vi "Model--Set Value.vi"(8 "error in":errorcluster, 10 "Value":i32, 11 "Selector in":refnum<class "Selector.lvclass">) -> (0 "error out":errorcluster, 3 "Selector out":refnum<class "Selector.lvclass">)   [LabVIEW 2019, in "Selector.lvclass"]
uses:
  Selector.lvclass
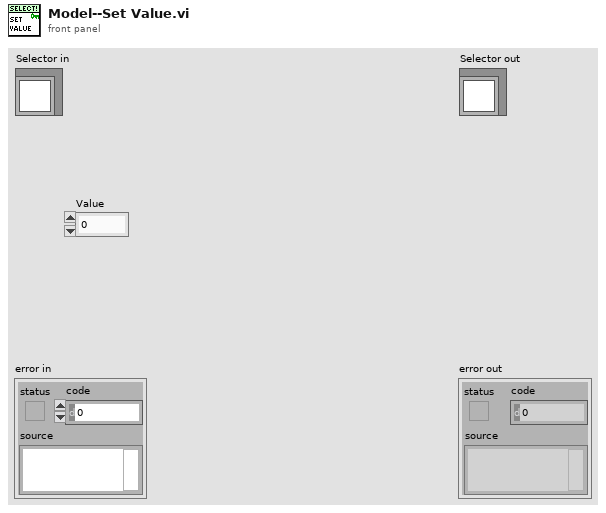
[diagram p1: front panel]
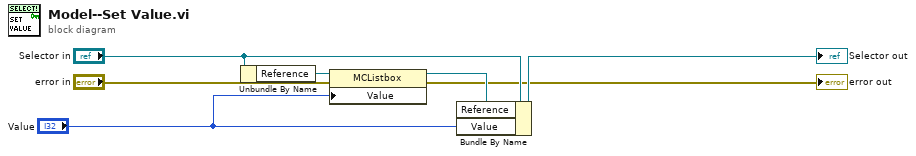
[diagram p0: block diagram]
diagram:
  n1 = Unbundle By Name("Selector in") -> ("Reference"=w7:refnum<vi>)
  n2 = property class="MCListbox"(reference=w7, error in="error in", "Value"="Value") -> (reference out=w3:refnum<vi>, error out=→"error out":errorcluster)
  n3 = Bundle By Name(cluster="Selector in", "Reference"=w3, "Value"="Value") -> (→"Selector out":refnum<class "Selector.lvclass">)
